vi "Write Registered Events.vi"(8 "error in (no error)":errorcluster, 10 "Reg Events":T1, 11 "Data Grid in":refnum<class "Data Grid.lvclass">) -> (0 "error out":errorcluster, 3 "Data Grid out":refnum<class "Data Grid.lvclass">)   [LabVIEW 2013, in "Table Manager.lvlib" / "Data Grid.lvclass"]
uses:
  Data Grid.lvclass
  <vilib>/DataGrid for LabVIEW/source/Events/Abstract EVENT/Abstract EVENT.lvclass
  <vilib>/NI/Configuration Framework/Node/StopEvent.ctl
  <vilib>/NI/Configuration Framework/Node/RefreshUIEvent.ctl
  <vilib>/NI/Configuration Framework/Node/CacheState.ctl
  <vilib>/NI/Configuration Framework/Node/NodeChangeEvent.ctl
  <vilib>/NI/Configuration Framework/Node/NodeRef.ctl
  <vilib>/NI/Configuration Framework/Node/NISE_CEF_Node.lvclass
  <vilib>/NI/Configuration Framework/Node/UserEventRef.ctl
  <vilib>/NI/Configuration Framework/Controls/EventCluster.ctl
  <vilib>/NI/DCAF/Tag Editor Core/control module/editor node/channel action event.ctl
  <vilib>/NI/DCAF/Tag Editor Core/control module/editor node/dialog output action.ctl
  <vilib>/NI/Tag Bus Module Framework/channel/TBM channel.lvclass
  <vilib>/NI/Tag Bus/tag/tag descriptor.lvclass
  Data Grid.lvclass/Data Grid.ctl
  <vilib>/NI/DCAF/Tag Editor Core/control module/editor node/control module editor.lvclass
  <vilib>/NI/Configuration Framework/NISE_CEF_TreeControl.lvlib
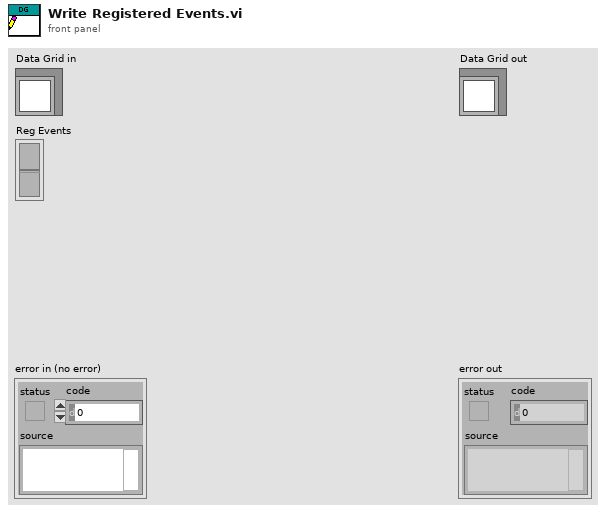
[diagram p1: front panel]
types:
  T1 = cluster{"Data Grid":refnum<event-registration>, "Node Events":refnum<event-registration>}
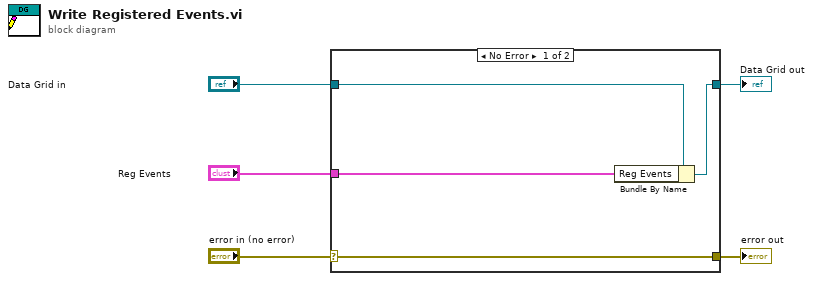
[diagram p0: block diagram]
diagram:
  n1 = case shown="No Error" "error in (no error)" {
    selector: "error in (no error)" -> [w9 w10]
    tunnel: [w9 w10] -> w4
    tunnel: [w7 w11] -> w2
    tunnel: "Data Grid in" -> [w8 w11]
    tunnel: "Reg Events" -> [w6 _]
    frame No Error {
      n2 = Bundle By Name(cluster=w8, "Reg Events"=w6) -> (w7:refnum<class "Data Grid.lvclass">)
    }
    frame Error {
    }
  }
  "error out" <- w4
  "Data Grid out" <- w2
